vi "accelerometer.vi"() -> ()   [LabVIEW 2017]
uses:
  <vilib>/LabVIEW Targets/FPGA/cRIO/shared/nicrio_ModuleControls/nicrio_cRIO-9232_ConfigModeRing.ctl
  <vilib>/LabVIEW Targets/FPGA/cRIO/shared/nicrio_ModuleControls/nicrio_cRIO-9230_DataRatesRing2.ctl
  <vilib>/rvi/Emulation/niFpgaGetClockAttributes.vi
  <vilib>/rvi/Emulation/niFpgaSctlEmulationGetInTimedLoop.vi
  <vilib>/rvi/Emulation/niFpgaEmulationReportErrorSimple.vi
  <vilib>/rvi/eio/common/nirviEmuTemplatePropertySet_errors.vi
  <vilib>/rvi/eio/common/nirviEmuTemplateMethod_errors.vi
  <vilib>/rvi/interface/RandomDataEmulation/niFpgaRandomDataHandleErrors.vi
  <vilib>/rvi/Emulation/niFpgaCriticalErrorInLSC.vi
  <vilib>/eio/EIOPropertyNode/EIOPropertyNode.xnode
  <vilib>/eio/EIONode/EIONode.xnode
  <vilib>/rvi/DataTransferAndStorage/Container/XNode/niFpgaContainer.xnode
  <vilib>/rvi/interface/RandomDataEmulation/nirviRandomDataFpgaReadWriteTemplate.vi
  <vilib>/eio/EIOMethodNode/EIOMethodNode.xnode
  <vilib>/rvi/eio/common/nirviEmuTemplatePropertyGet_errors.vi
  <vilib>/rvi/eio/common/nirviEmuTemplatePropertyGet_noerrors.vi
  <vilib>/rvi/eio/common/nirviEmuTemplatePropertySet_noerrors.vi
panel:
  in  "Data Rate":T1=10 items=["12.800 kS/s (NI 9230)"=10, "11.378 kS/s (NI 9230)"=36, "10.240 kS/s (NI 9230)"=21, "9.309 kS/s (NI 9230)"=44, "8.533 kS/s (NI 9230)"=14, "7.877 kS/s (NI 9230)"=52, "7.314 kS/s (NI 9230)"=29, "6.827 kS/s (NI 9230)"=60, "6.400 kS/s (NI 9230)"=18, "6.024 kS/s (NI 9230)"=68, "5.689 kS/s (NI 9230)"=37, "5.389 kS/s (NI 9230)"=76, "5.120 kS/s (NI 9230)"=22, "4.876 kS/s (NI 9230)"=84, "4.655 kS/s (NI 9230)"=45, "4.452 kS/s (NI 9230)"=92, "4.267 kS/s (NI 9230)"=26, "4.096 kS/s (NI 9230)"=100, "3.938 kS/s (NI 9230)"=53, "3.657 kS/s (NI 9230)"=30, "3.413 kS/s (NI 9230)"=61, "3.200 kS/s (NI 9230)"=34, "3.012 kS/s (NI 9230)"=69, "2.844 kS/s (NI 9230)"=38, "2.695 kS/s (NI 9230)"=77, "2.560 kS/s (NI 9230)"=42, "2.438 kS/s (NI 9230)"=85, "2.327 kS/s (NI 9230)"=46, "2.226 kS/s (NI 9230)"=93, "2.133 kS/s (NI 9230)"=50, "2.048 kS/s (NI 9230)"=101, "1.969 kS/s (NI 9230)"=54, "1.829 kS/s (NI 9230)"=58, "1.707 kS/s (NI 9230)"=62, "1.600 kS/s (NI 9230)"=66, "1.506 kS/s (NI 9230)"=70, "1.422 kS/s (NI 9230)"=74, "1.347 kS/s (NI 9230)"=78, "1.280 kS/s (NI 9230)"=82, "1.219 kS/s (NI 9230)"=86, "1.164 kS/s (NI 9230)"=90, "1.113 kS/s (NI 9230)"=94, "1.067 kS/s (NI 9230)"=98, "1.024 kS/s (NI 9230)"=102, "0.985 kS/s (NI 9230)"=106]
  out "Open Loop":bool[](array[boolean])
  out "Short Circuit":bool[](array[boolean])
  out "Data FIFO Full":bool
  out "Error Out":errorcluster
  in  "Input Configuration":T2=2 items=["AC Coupled", "DC Coupled", "IEPE AC Coupled"]
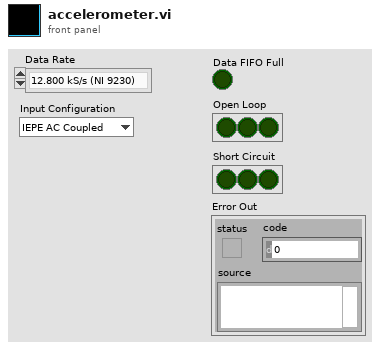
[diagram p1: front panel]
types:
  T1 = typedef "nicrio_cRIO-9230_DataRatesRing2.ctl" = u8
  T2 = typedef "nicrio_cRIO-9232_ConfigModeRing.ctl" = u8
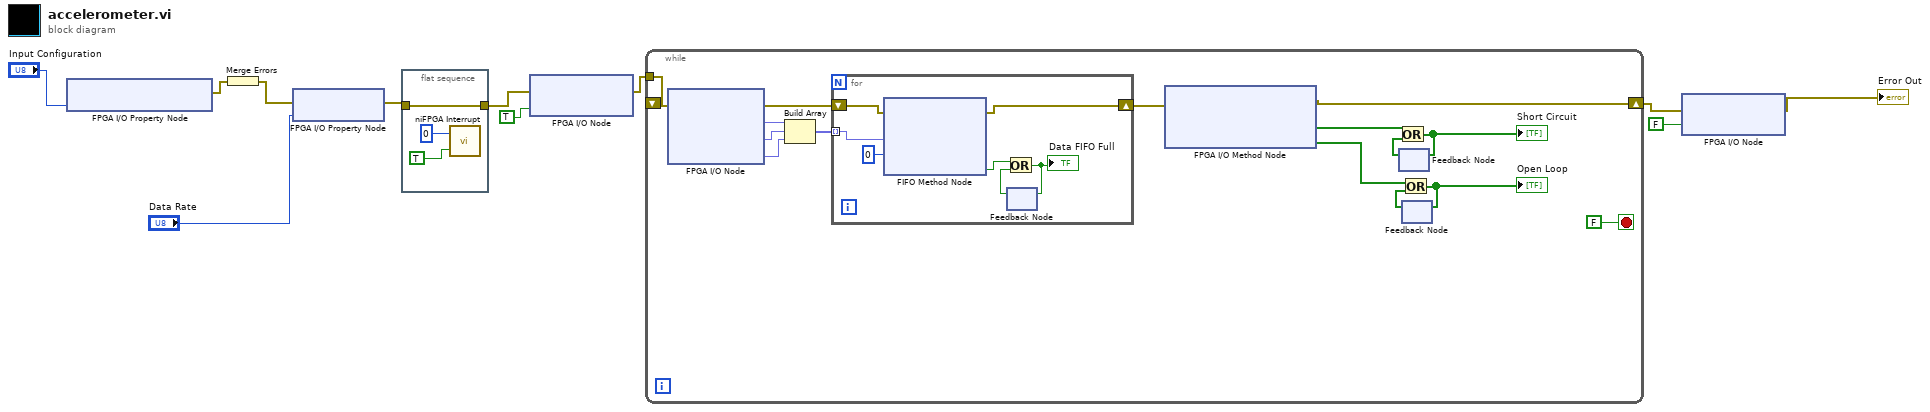
[diagram p0: block diagram]
diagram:
  n1 = xnode "FPGA I/O Property Node"("Input Configuration"="Input Configuration") -> ("error out"=w10:errorcluster)  [unwired: 2 in, 1 out]
  n2 = Merge Errors(w10) -> (w9:errorcluster)
  n3 = xnode "FPGA I/O Property Node"("error in"=w9, "Data Rate"="Data Rate") -> ("error out"=w7:errorcluster)  [unwired: 1 in, 1 out]
  n4 = flat-sequence {
    tunnel: [w12] -> w6
    tunnel: w7 -> [w12]
    frame #0 {
      n5 = call <vilib>:"niFPGA Interrupt.vi"("Wait Until Cleared (F)"=TRUE ("Wait Until Cleared"), "IRQ Number (0)"=u8 0 ("IRQ Bit (0-31)")) -> ()  [unwired: 1 in]
    }
  }
  n6 = xnode "FPGA I/O Node"("error in"=w6, "Mod8/Start"=TRUE) -> ("error out"=w5:errorcluster)  [unwired: 1 in, 1 out]
  n7 = while {
    shift-right: [w18] -> w3
    shift-left: _ -> [_]
    tunnel: w5 -> [w22]
    stop <- FALSE stop-if-true
    n8 = xnode "FPGA I/O Node"("error in"=w22) -> ("error out"=w27:errorcluster, "Mod8/AI0"=w29:fxp<+/-,24,7>, "Mod8/AI1"=w16:fxp<+/-,24,7>, "Mod8/AI2"=w15:fxp<+/-,24,7>)  [unwired: 3 in, 3 out]
    n9 = Build Array(w29, w16, w15) -> (w28:fxp<+/-,24,7>[])
    n10 = for {
      tunnel: w28 -> [w32] mode=indexing
      shift-right: [w33] -> w21
      shift-left: w27 -> [w34]
      n11 = xnode ("FIFO Method Node")("Element"=w32, "Timeout"=0, "error in (no error)"=w34) -> ("Timed Out?"=w30:bool, "error out"=w33:errorcluster)  [unwired: 1 in, 1 out]
      n12 = feedback #1() -> (w35:bool)  [unwired: 1 out]
      n13 = Or(x=w30, y=w35) -> (x .or. y?=w36:bool)
      "Data FIFO Full" <- w36
      n14 = feedback-in #1(w36) -> ()
    }
    n15 = xnode "FPGA I/O Method Node"("error in"=w21) -> ("error out"=w18:errorcluster, "Short Circuit"=w20:bool[], "Open Loop"=w19:bool[])  [unwired: 1 in, 1 out]
    n16 = feedback #2() -> (w24:bool[])  [unwired: 1 out]
    n17 = Or(x=w20, y=w24) -> (x .or. y?=w23:bool[])
    "Short Circuit" <- w23
    n18 = feedback-in #2(w23) -> ()
    n19 = feedback #3() -> (w26:bool[])  [unwired: 1 out]
    n20 = Or(x=w19, y=w26) -> (x .or. y?=w25:bool[])
    "Open Loop" <- w25
    n21 = feedback-in #3(w25) -> ()
  }
  n22 = xnode "FPGA I/O Node"("error in"=w3, "Mod8/Stop"=FALSE) -> ("error out"=→"Error Out":errorcluster)  [unwired: 1 in, 1 out]
